vi "Test Process No Process Errors Through Basic Lifecycle.vi"(8 "error in (no error)":errorcluster, 11 "Process Test In":refnum<class "Process Test.lvclass">) -> (0 "error out":errorcluster, 3 "Process Test Out":refnum<class "Process Test.lvclass">)   [LabVIEW 2020, in "Process Test.lvclass"]
uses:
  Process Test.lvclass
  C:/Program Files (x86)/National Instruments/LabVIEW 2020/vi.lib/Asteme/LUnit/Test Case.lvclass
  Mock Error Handler/Mock Error Handler.lvclass
  C:/Users/anton/Documents/GitHub/Triarc-Framework/source/Framework/Process/Process.lvclass
  C:/Users/anton/Documents/GitHub/Triarc-Framework/source/Framework/Error Handler Interface/Error Handler Interface.lvclass
  Framework/Process/Process.lvclass/Process.ctl
  <vilib>/Asteme/LUnit/Test Case.lvclass/Test Case.ctl
  <vilib>/Asteme/LUnit/LUnit Assertion Result.lvclass/LUnit Assertion Result.ctl
  Framework/Process/Public/Get Lifecycle State.vi
  Framework/Process/Protected/Messaging/Enqueue Message.vi
  <vilib>/Utility/error.llb/Clear Errors.vi
  Framework/Process/Private/SubVIs/Wait for finish.vi
  Framework/Process/Private/SubVIs/Set Lifecycle State.vi
  <vilib>/Asteme/LUnit/Palette/Pass.vi
  <vilib>/Asteme/LUnit/Palette/Fail.vi
  <vilib>/Asteme/LUnit/Set Assertion Type.vi
  <vilib>/AdvancedString/1D String Array to Delimited String.vi
  <vilib>/Asteme/LUnit/Add test result.vi
  <vilib>/Asteme/LUnit/LUnit Write Passed.vi
  <vilib>/Asteme/LUnit/LUnit Get Test Case.vi
  <vilib>/Asteme/LUnit/LUnit Write Message.vi
  <vilib>/Asteme/LUnit/LUnit Write Description.vi
  <vilib>/Asteme/LUnit/LUnit Write Assertion Type.vi
  <vilib>/Asteme/LUnit/Read Test Case Name.vi
  <vilib>/Utility/error.llb/Error Cluster From Error Code.vi
  <vilib>/Asteme/LUnit/Assertion Result/LUnit Get Test Name.vi
  Framework/Process/Process.lvclass
  <vilib>/Asteme/LUnit/LUnit Assertion Result.lvclass
  <vilib>/Asteme/LUnit/Test Case.lvclass
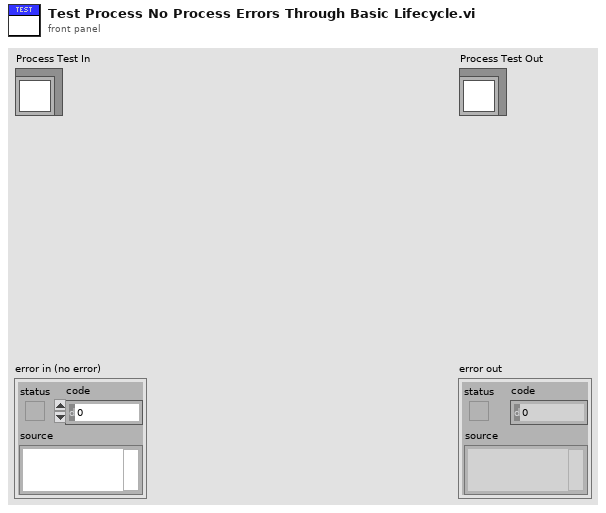
[diagram p1: front panel]
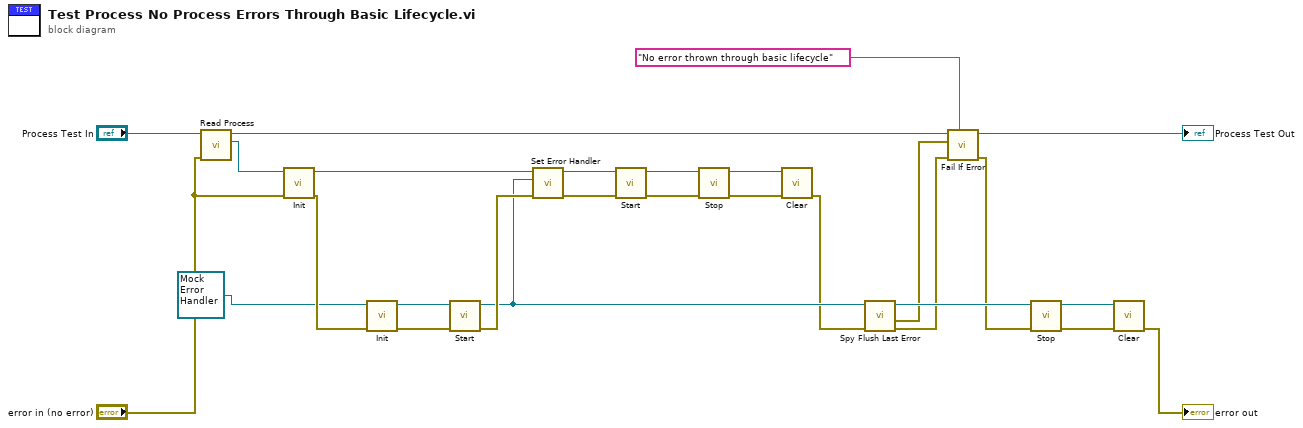
[diagram p0: block diagram]
diagram:
  n1 = call "Read Process.vi"("error in (no error)"="error in (no error)", "Process Test in"="Process Test In") -> ("Process.lvclass"=w4:refnum<class "Process.lvclass">, "Process Test out"=w3:refnum<class "Process Test.lvclass">)  [unwired: 7 in, 1 out]
  n2 = call-dynamic "Init.vi"("error in (no error)"="error in (no error)", "Process In"=w4) -> ("error out"=w26:errorcluster, "Process Out"=w23:refnum<class "Process.lvclass">)  [unwired: 8 in]
  n3 = call-dynamic "Init.vi"("error in (no error)"=w26, "Mock Error Handler In"=refnum<class "Mock Error Handler.lvclass"> refnum ("Mock Error Handler.lvclass")) -> ("error out"=w15:errorcluster, "Mock Error Handler Out"=w16:refnum<class "Mock Error Handler.lvclass">)  [unwired: 8 in]
  n4 = call "Start.vi"("error in (no error)"=w15, "Process In"=w16) -> ("error out"=w25:errorcluster, "Process Out"=w10:refnum<class "Mock Error Handler.lvclass">)  [unwired: 8 in]
  n5 = call "Set Error Handler.vi"("error in (no error)"=w25, "Error Handler"=w10, "Process In"=w23) -> ("error out"=w21:errorcluster, "Process Out"=w22:refnum<class "Process.lvclass">)  [unwired: 7 in]
  n6 = call "Start.vi"("error in (no error)"=w21, "Process In"=w22) -> ("error out"=w19:errorcluster, "Process Out"=w20:refnum<class "Process.lvclass">)  [unwired: 8 in]
  n7 = call "Stop.vi"("error in (no error)"=w19, "Process In"=w20) -> ("error out"=w17:errorcluster, "Process Out"=w18:refnum<class "Process.lvclass">)  [unwired: 7 in, 1 out]
  n8 = call-dynamic "Clear.vi"("error in (no error)"=w17, "Process In"=w18) -> ("error out"=w9:errorcluster)  [unwired: 8 in, 1 out]
  n9 = call "Spy Flush Last Error.vi"("error in (no error)"=w9, "Mock Error Handler In"=w10) -> ("error out"=w8:errorcluster, "Errors"=w7:errorcluster, "Mock Error Handler Out"=w14:refnum<class "Mock Error Handler.lvclass">)  [unwired: 6 in, 1 out]
  n10 = call <vilib>:"Fail If Error.vi"("Description"="No error thrown through basic lifecycle", "error in (no error)"=w8, "Assert error"=w7, "Test Case In"=w3) -> ("error out"=w6:errorcluster, "Test Case Out"=→"Process Test Out":refnum<class "Process Test.lvclass">)  [unwired: 6 in]
  n11 = call "Stop.vi"("error in (no error)"=w6, "Process In"=w14) -> ("error out"=w12:errorcluster, "Process Out"=w13:refnum<class "Mock Error Handler.lvclass">)  [unwired: 7 in, 1 out]
  n12 = call-dynamic "Clear.vi"("error in (no error)"=w12, "Process In"=w13) -> ("error out"=→"error out":errorcluster)  [unwired: 8 in, 1 out]
